vi "YFM최종.vi"() -> ()   [LabVIEW 2017]
uses:
  <vilib>/DAQmx/create/channels.llb/DAQmx Create Channel (AO-Voltage-Basic).vi
  <vilib>/DAQmx/configure/timing.llb/DAQmx Timing (Sample Clock).vi
  <vilib>/DAQmx/create/channels.llb/DAQmx Create Channel (AI-Voltage-Basic).vi
  <vilib>/DAQmx/write.llb/DAQmx Write (Analog Wfm 1Chan NSamp).vi
panel:
  in  "rate":dbl=1000.0 format="%0.2f"
  in  "Vd channel":tag
  in  "Vg channel":tag
  in  "Id channel":tag
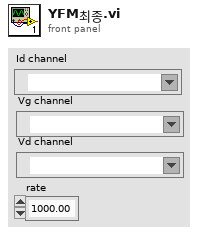
[diagram p1: front panel]
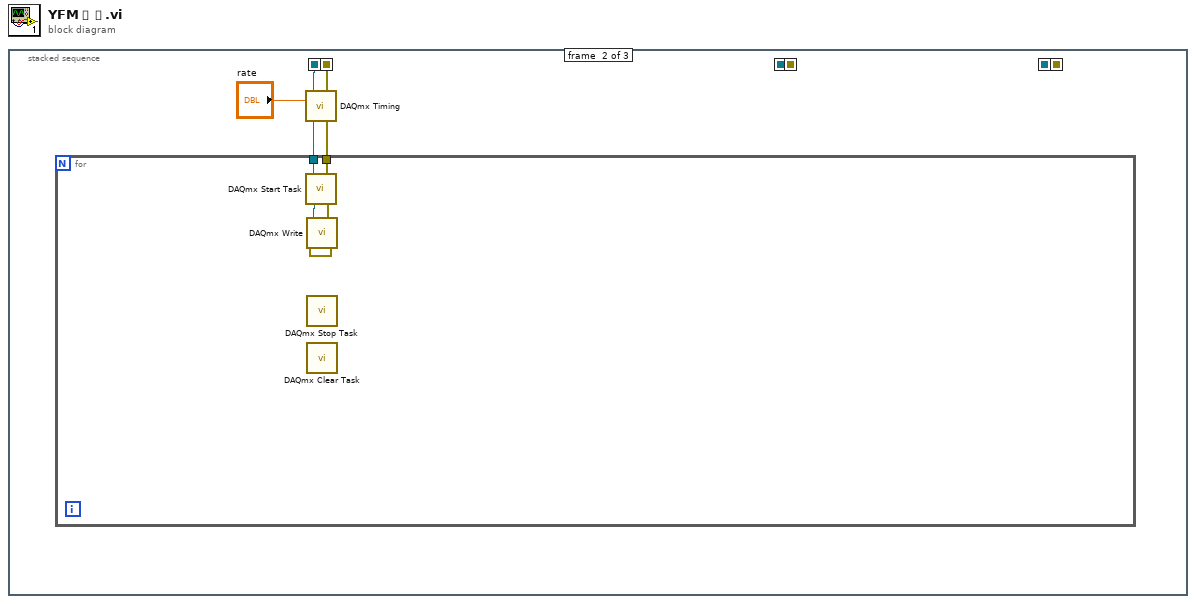
[diagram p0: block diagram]
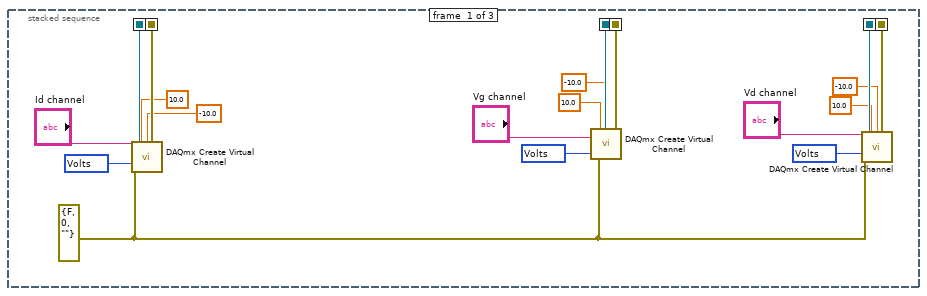
[diagram p2: hidden frame]
diagram:
  n1 = stacked-sequence {
    seq-local: [w19 _ _] -> [_ w24 _]
    seq-local: [w18 _ _] -> [_ w23 _]
    seq-local: [w11 _ _] -> [_ _ _]
    seq-local: [w10 _ _] -> [_ _ _]
    seq-local: [w9 _ _] -> [_ _ _]
    seq-local: [w8 _ _] -> [_ _ _]
    frame #0 {
      w1 = 10348 items=["Volts"=10348, "From Custom Scale"=10065] ("units")
      w2 = 10348 items=["Volts"=10348, "From Custom Scale"=10065] ("units")
      w7 = errorcluster {"status"=FALSE, "code"=0, "source"=""} ("error in")
      w14 = 10348 items=["Volts"=10348, "From Custom Scale"=10065] ("units")
      n2 = call-poly <vilib>:"DAQmx Create Virtual Channel.vi"("maximum value"=10.0, "minimum value"=-10.0, "physical channels"="Id channel", "units"=w14, "error in"=w7) -> ("task out"=w19:refnum<k21>, "error out"=w18:errorcluster)  [unwired: 9 in]
      n3 = call-poly <vilib>:"DAQmx Create Virtual Channel.vi"("maximum value"=10.0, "minimum value"=-10.0, "physical channels"="Vg channel", "units"=w2, "error in"=w7) -> ("task out"=w11:refnum<k21>, "error out"=w10:errorcluster)  [unwired: 9 in]
      n4 = call-poly <vilib>:"DAQmx Create Virtual Channel.vi"("maximum value"=10.0, "minimum value"=-10.0, "physical channels"="Vd channel", "units"=w1, "error in"=w7) -> ("task out"=w9:refnum<k21>, "error out"=w8:errorcluster)  [unwired: 9 in]
    }
    frame #1 {
      n5 = call-poly <vilib>:"DAQmx Timing.vi"("task/channels in"=w24, "rate"="rate", "error in"=w23) -> ("task out"=w21:refnum<k21>, "error out"=w20:errorcluster)  [unwired: 11 in]
      n6 = for {
        tunnel: w21 -> [w28]
        tunnel: w20 -> [w27]
        n7 = call <vilib>:"DAQmx Start Task.vi"("task/channels in"=w28, "error in"=w27) -> ("task out"=w26:refnum<k21>, "error out"=w25:errorcluster)  [unwired: 12 in]
        n8 = call-poly <vilib>:"DAQmx Write.vi"("task/channels in"=w26, "error in"=w25) -> ()  [unwired: 11 in, 3 out]
        n9 = call <vilib>:"DAQmx Stop Task.vi"() -> ()  [unwired: 14 in, 2 out]
        n10 = call <vilib>:"DAQmx Clear Task.vi"() -> ()  [unwired: 15 in, 1 out]
      }
    }
    frame #2 {
    }
  }
